vi "De-Initialize.vi"(8 "error in (no error)":errorcluster, 11 "Quantum Design Driver in":refnum<class "Quantum Design Driver.lvclass">) -> (0 "error out":errorcluster, 3 "Quantum Design Driver out":refnum<class "Quantum Design Driver.lvclass">)   [LabVIEW 2018, in "Quantum Design Driver.lvclass"]
uses:
  Quantum Design Driver.lvclass
  Quantum Design Driver.lvclass/Quantum Design Driver.ctl
  Simple VISA Reader/Simple VISA Reader Driver.lvclass
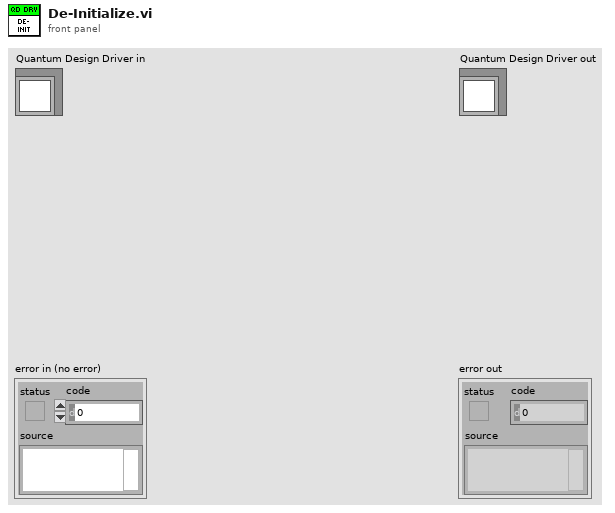
[diagram p1: front panel]
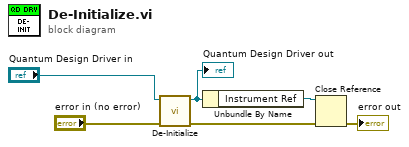
[diagram p0: block diagram]
diagram:
  n1 = call-parent "De-Initialize.vi"("error in (no error)"="error in (no error)", "Instrument Driver in"="Quantum Design Driver in") -> ("error out"=w2:errorcluster, "Instrument Driver out"=w4:refnum<class "Quantum Design Driver.lvclass">)  [unwired: 8 in]
  "Quantum Design Driver out" <- w4
  n2 = Unbundle By Name(w4) -> ("Instrument Ref"=w3:refnum<k24>)
  n3 = Close Reference(reference=w3, error in (no error)=w2) -> (error out=→"error out":errorcluster)
